vi "CRYRead Config Settings.vi"(8 "error in (no error)":errorcluster, 10 "Section":string[](array[string])) -> (0 "error out":errorcluster, 2 "Configuration Data":T1(array[cluster]))   [LabVIEW 2013]
doc: "Illustrates how to read a configuration settings file.\n\nInstructions:\nRun Write Configuration Settings File.vi, located in the file\\config.llb. Then run this VI and select the appropriate configuration settings file to load."
uses:
  CRYMainGlobal.vi
  <vilib>/Utility/config.llb/Read Key (String).vi
  <vilib>/Utility/config.llb/NI_LVConfig.lvlib
panel:
  in  "Config Data":T2
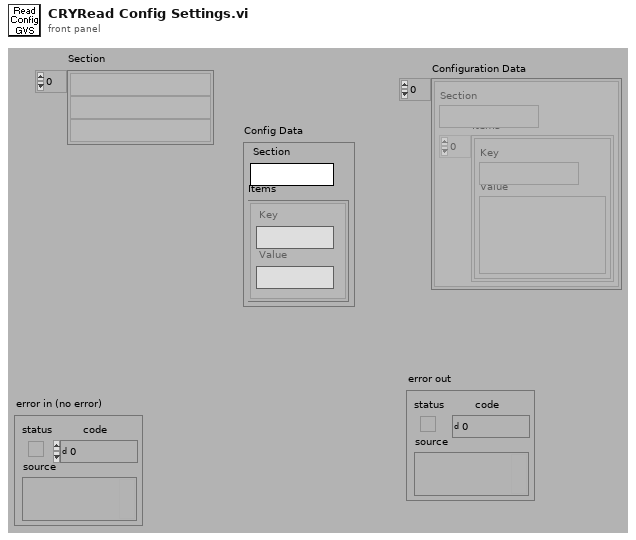
[diagram p1: front panel]
types:
  T1 = cluster{"Section":string, "Items":cluster{"Key":string, "Value":string}[]}[]
  T2 = cluster{"Section":string, "Items":cluster{"Key":string, "Value":string}[]}
  T3 = typedef "NI_LVConfig.lvlib/Config Data RefNum.ctl" = refnum<k1>
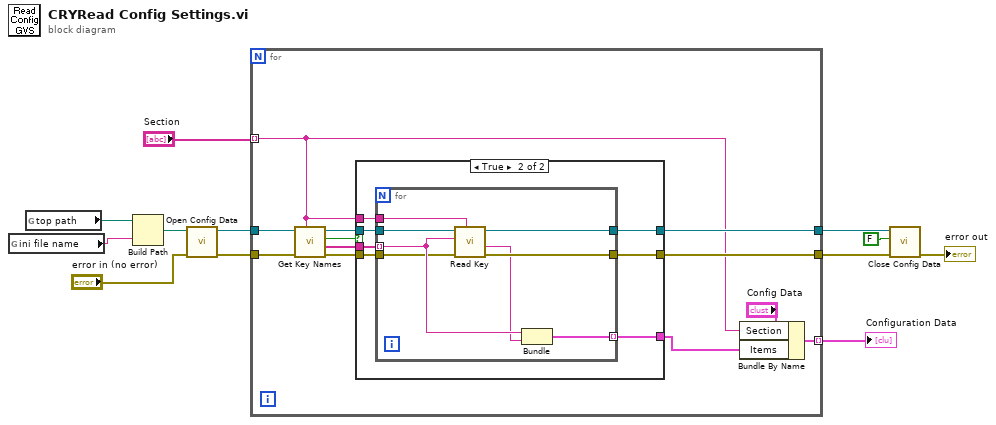
[diagram p0: block diagram]
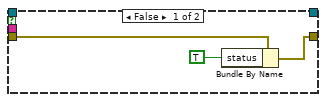
[diagram p2: hidden frame]
diagram:
  n1 = global read "CRYMainGlobal.vi" "ini file name"() -> (w7:string)
  n2 = global read "CRYMainGlobal.vi" "top path"() -> (w9:path)
  n3 = Build Path(base path=w9, name or relative path=w7) -> (appended path=w4:path)
  n4 = call <vilib>:"Open Config Data.vi"("error in (no error)"="error in (no error)", "configuration file path"=w4) -> ("error out"=w1:errorcluster, "refnum"=w2:T3)  [unwired: 7 in, 1 out]
  n5 = for {
    tunnel: w2 -> [w24]
    tunnel: [w20] -> w11
    tunnel: [w19] -> w10
    tunnel: w1 -> [w17]
    tunnel: "Section" -> [w16] mode=indexing
    tunnel: [w14] -> w5 mode=indexing
    n6 = call <vilib>:"Get Key Names.vi"("section"=w16, "error in (no error)"=w17, "refnum"=w24) -> ("error out"=w18:errorcluster, "key names"=w21:string[], "section exists?"=w23:bool, "refnum out"=w22:T3)  [unwired: 5 out]
    n7 = case shown="True" w23 {
      tunnel: w22 -> [_ w33]
      tunnel: w21 -> [_ w34]
      tunnel: [_ w32] -> w20
      tunnel: [w25 w31] -> w19
      tunnel: [_ w30] -> w15
      tunnel: w18 -> [w27 w29]
      tunnel: w16 -> [_ w28]
      frame False {
        n8 = Bundle By Name(cluster=w27, "status"=TRUE) -> (w25:errorcluster)
      }
      frame True {
        n9 = for {
          tunnel: w34 -> [w39] mode=indexing
          tunnel: w33 -> [w42]
          tunnel: [w41] -> w32
          tunnel: [w40] -> w31
          tunnel: [w37] -> w30 mode=indexing
          tunnel: w29 -> [w36]
          tunnel: w28 -> [w35]
          n10 = call-poly <vilib>:"Read Key.vi"("section"=w35, "error in (no error)"=w36, "key"=w39, "refnum"=w42) -> ("error out"=w40:errorcluster, "value"=w38:string, "refnum out"=w41:T3)  [unwired: 2 in, 3 out]
          n11 = Bundle("String"=w39, "value"=w38) -> (w37:cluster{"String":string, "value":string})  [unwired: 1 out]
        }
      }
    }
    n12 = Bundle By Name(cluster="Config Data", "Section"=w16, "Items"=w15) -> (w14:T2)
  }
  "Configuration Data" <- w5
  n13 = call <vilib>:"Close Config Data.vi"("error in (no error)"=w10, "write file if changed (T)"=FALSE ("write configuration file? (T)"), "refnum"=w11) -> ("error out"=→"error out":errorcluster)  [unwired: 8 out]
